vi "Report.vi"(6 "文件重命名":bool, 7 "文件名称":string, 8 "错误输入（无错误）":errorcluster) -> (0 "error out":errorcluster caption="错误输出")   [LabVIEW 2020]
uses:
  Database/Global1.vi
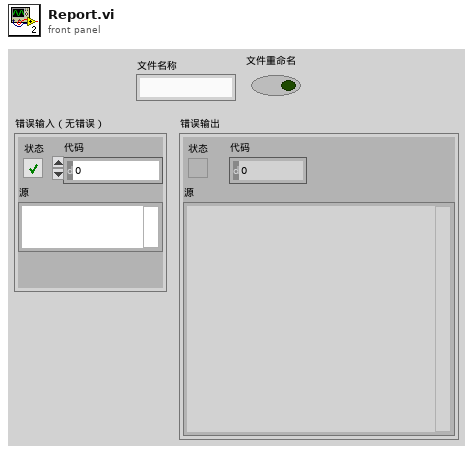
[diagram p1: front panel]
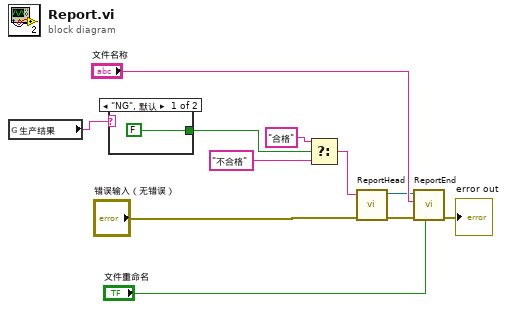
[diagram p0: block diagram]
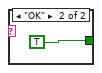
[diagram p2: hidden frame]
diagram:
  n1 = global read "Global1.vi" "生产结果"() -> (w2:string)
  n2 = case shown="\"NG\", 默认" w2 {
    tunnel: [FALSE TRUE] -> w1
    frame "NG", Default {
    }
    frame "OK" {
    }
  }
  n3 = Select(t="合格", s=w1, f="不合格") -> (s? t:f=w6:string)
  n4 = call "ReportHead.vi"("error in (no error)"="错误输入（无错误）", "产品状态"=w6) -> ("error out"=w3:errorcluster, "report out"=w4:refnum<class "NI_report.lvclass">)  [unwired: 8 in]
  n5 = call "ReportEnd.vi"("文件重命名"="文件重命名", "error in (no error)"=w3, "文件名称"="文件名称", "report in"=w4) -> ("error out"=→"error out":errorcluster)  [unwired: 7 in]
